vi "PFI-28000-Utils_Check Command Reply.vi"(0 "Command":string, 5 "Reply":string, 11 "error in (no error)":errorcluster) -> (15 "error out":errorcluster)   [LabVIEW 2017, in "PFI-28000-Utils.lvlib"]
uses:
  PFI-28000-Utils.lvlib
  <vilib>/regexp/Match Regular Expression.xnode
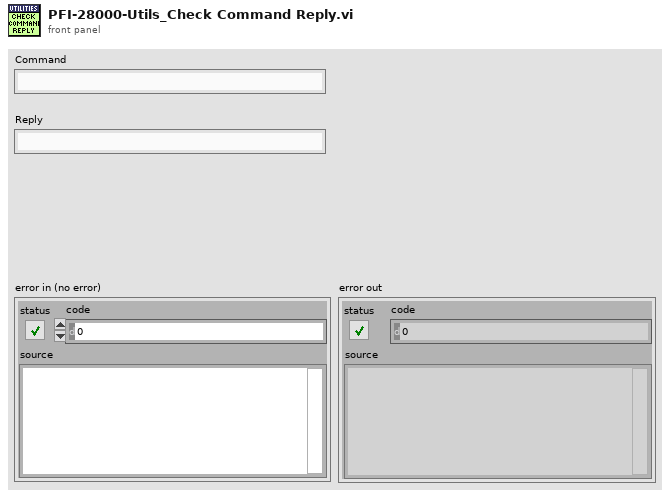
[diagram p1: front panel]
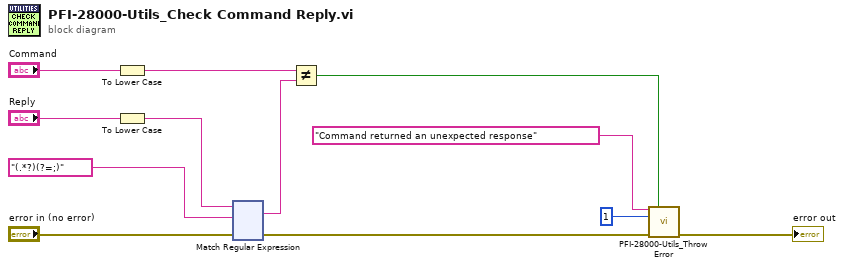
[diagram p0: block diagram]
diagram:
  n1 = To Lower Case(string="Command") -> (all lower case string=w2:string)
  n2 = To Lower Case(string="Reply") -> (all lower case string=w1:string)
  n3 = xnode "Match Regular Expression"("input string"=w1, "regular expression"="(.*?)(?=;)" ("empty string"), "error in"="error in (no error)") -> ("whole match"=w8:string, "error out"=w7:errorcluster)  [unwired: 3 in, 3 out]
  n4 = Not Equal?(x=w2, y=w8) -> (x != y?=w6:bool)
  n5 = call "PFI-28000-Utils_Throw Error.vi"("Error Message"="Command returned an unexpected response" ("empty string"), "Throw?"=w6, "Error Code"=1, "error in (no error)"=w7) -> ("error out"=→"error out":errorcluster)  [unwired: 11 in]
